vi "Test Gantry Camera.vi"() -> ()   [LabVIEW 2011]
uses:
  Type Definitions/Gantry_Camera.ctl
  <vilib>/userdefined/High Color/IMAQdx.ctl
  Gantry Class.lvclass
panel:
  out "Cameras":T1[](array[typedef])
  out "Gantry Head":T3(plugin-control)
  in  "Config Folder":path=path "C:/Users/Husker/Desktop/gantry/Config"
  out "Needle Calibration 2":T3(plugin-control)
  out "error out":errorcluster {"code" format="%.0x"}
  out "Needle Calibration 1":T3(plugin-control)
  in  "stop":bool
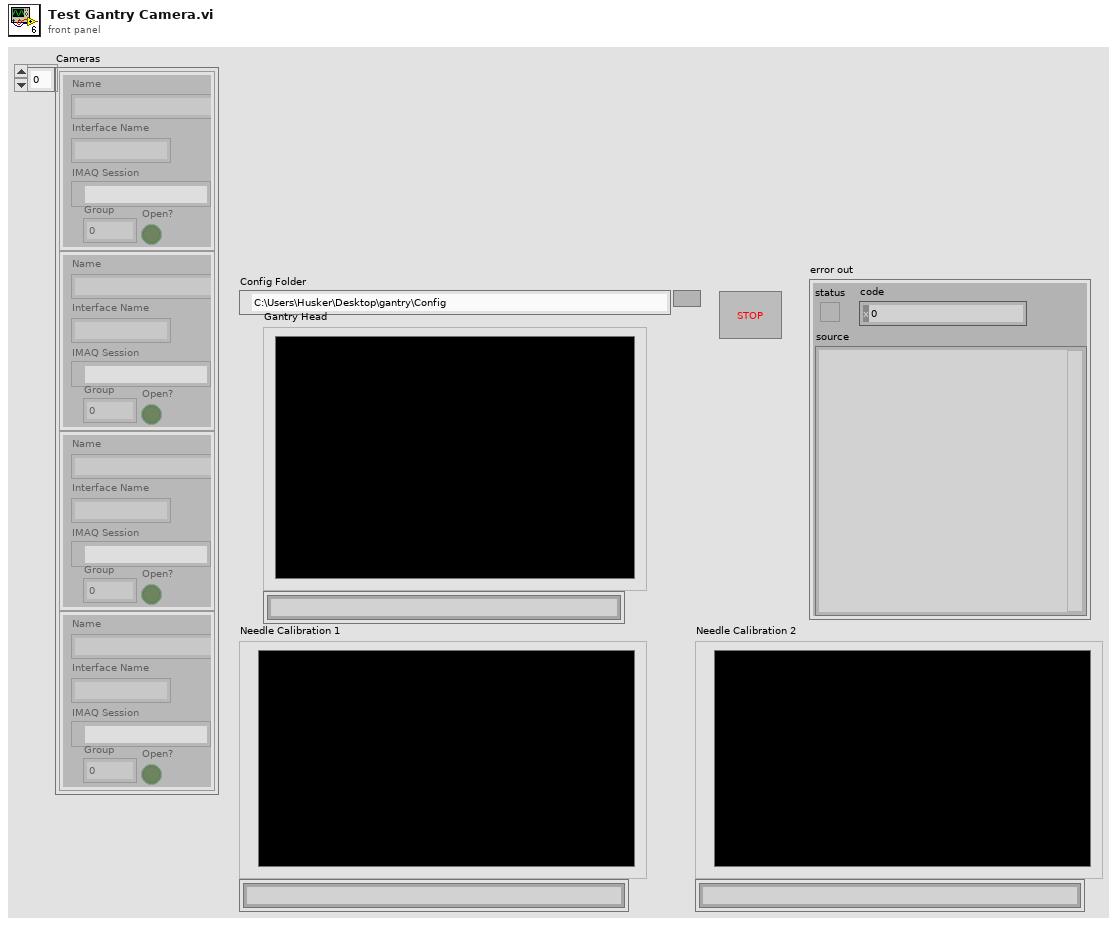
[diagram p1: front panel]
types:
  T1 = typedef "Gantry_Camera.ctl" = cluster{"Name":string, "IMAQ Session":T2, "Group":u32, "Open?":bool, "Interface Name":string}
  T2 = typedef "IMAQdx.ctl" = refnum<k21>
  T3 = typedef "IMAQ Image.ctl" = refnum<image>
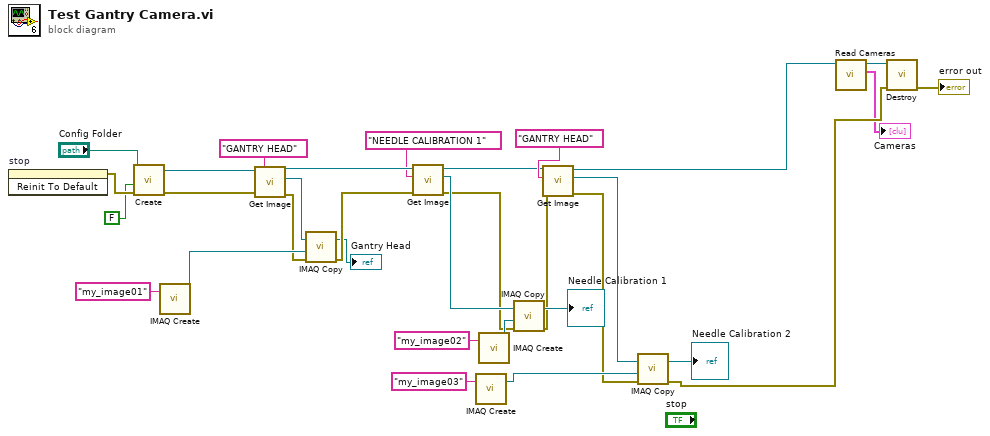
[diagram p0: block diagram]
diagram:
  n1 = invoke on="stop" class="Bool (strict)" method="Reinit To Default"() -> (error out=w26:errorcluster)  [unwired: 3 in, 2 out]
  n2 = call "Create.vi"("error in (no error)"=w26, "HOME?"=FALSE, "Config Folder"="Config Folder") -> ("error out"=w31:errorcluster, "Gantry Class out"=w32:refnum<class "Gantry Class.lvclass">)  [unwired: 7 in]
  n3 = call "IMAQ Create"("Image Name"="my_image01") -> ("New Image"=w29:T3)  [unwired: 4 in, 1 out]
  n4 = call "Get Image.vi"("error in (no error)"=w31, "Camera Name"="GANTRY HEAD", "Gantry Class in"=w32) -> ("error out"=w22:errorcluster, "Image Out"=w24:T3, "Gantry Class out"=w23:refnum<class "Gantry Class.lvclass">)  [unwired: 6 in]
  n5 = call "IMAQ Copy"("error in (no error)"=w22, "Image Dst"=w29, "Image Src"=w24) -> ("error out"=w21:errorcluster, "Image Dst Out"=→"Gantry Head":T3)  [unwired: 3 in]
  n6 = call "Get Image.vi"("error in (no error)"=w21, "Camera Name"="NEEDLE CALIBRATION 1", "Gantry Class in"=w23) -> ("error out"=w4:errorcluster, "Image Out"=w10:T3, "Gantry Class out"=w7:refnum<class "Gantry Class.lvclass">)  [unwired: 6 in]
  n7 = call "IMAQ Create"("Image Name"="my_image03") -> ("New Image"=w12:T3)  [unwired: 4 in, 1 out]
  n8 = call "IMAQ Create"("Image Name"="my_image02") -> ("New Image"=w14:T3)  [unwired: 4 in, 1 out]
  n9 = call "IMAQ Copy"("error in (no error)"=w4, "Image Dst"=w14, "Image Src"=w10) -> ("error out"=w3:errorcluster, "Image Dst Out"=→"Needle Calibration 1":T3)  [unwired: 3 in]
  n10 = call "Get Image.vi"("error in (no error)"=w3, "Camera Name"="GANTRY HEAD", "Gantry Class in"=w7) -> ("error out"=w2:errorcluster, "Image Out"=w5:T3, "Gantry Class out"=w19:refnum<class "Gantry Class.lvclass">)  [unwired: 6 in]
  n11 = call "IMAQ Copy"("error in (no error)"=w2, "Image Dst"=w12, "Image Src"=w5) -> ("error out"=w28:errorcluster, "Image Dst Out"=→"Needle Calibration 2":T3)  [unwired: 3 in]
  n12 = call-dynamic "Read Cameras.vi"("Gantry Class in"=w19) -> ("Cameras"=→"Cameras":T1[], "Gantry Class out"=w18:refnum<class "Gantry Class.lvclass">)  [unwired: 8 in, 1 out]
  n13 = call "Destroy.vi"("error in (no error)"=w28, "Gantry Class in"=w18) -> ("error out"=→"error out":errorcluster)  [unwired: 9 in]
